vi "数据存储.vi"(10 "字符串":string="E:\\YM\\", 11 "2D data":dbl[][](array[numeric]) caption="二维数据" format="%0.2f") -> ()   [LabVIEW 2013]
uses:
  <vilib>/printing/EasyPrintingControls.llb/report_type.ctl
  <vilib>/printing/EasyPrintingControls.llb/contents.ctl
  <vilib>/Utility/NIReport.llb/NI_report.lvclass
  <vilib>/Utility/file.llb/Write To Spreadsheet File (DBL).vi
  <vilib>/printing/EasyPrinting.llb/Easy Print VI Panel or Documentation (path).vi
  <vilib>/Utility/NIReport.llb/NI_ReportGenerationCore.lvlib
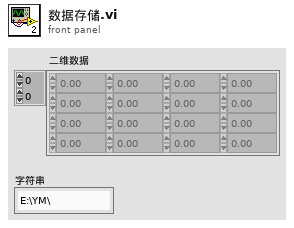
[diagram p1: front panel]
types:
  T1 = typedef "NI_ReportGenerationCore.lvlib/contents.ctl" = u16
  T2 = typedef "NI_ReportGenerationCore.lvlib/report_type.ctl" = u16
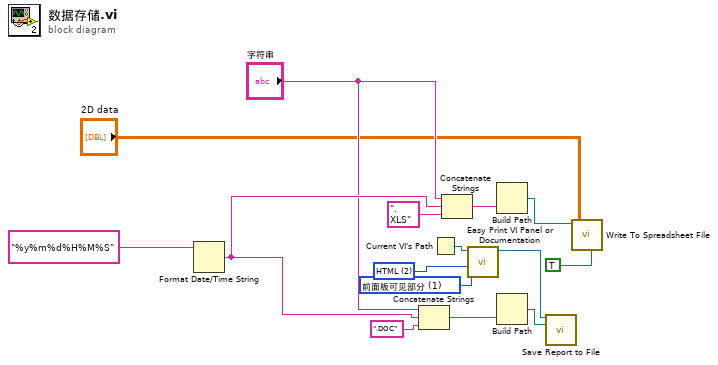
[diagram p0: block diagram]
diagram:
  w3 = T1 1 items=["完整前面板", "前面板可见部分", "图标、说明、前面板和程序框图", "说明信息：使用前面板", "说明信息：作为子VI使用", "说明信息：完整", "说明信息：自定义"] ("contents (complete front panel)")
  w11 = T2 2 items=["快速打印", "标准报表", "HTML", "双字节", "Excel"] ("report type (Quick Print)")
  n1 = Format Date/Time String(time format string (%c)="%y%m%d%H%M%S" ("时间格式字符串(%c)")) -> (date/time string=w6:string)  [unwired: 2 in]
  n2 = Concatenate Strings("字符串", w6, ".DOC" ("产品ID")) -> (w9:string)
  n3 = Current VI's Path() -> (path=w12:path)
  n4 = Concatenate Strings("字符串", w6, ".XLS") -> (w14:string)
  n5 = call-poly <vilib>:"Easy Print VI Panel or Documentation.vi"("report type (Quick Print)"=w11, "contents (complete front panel)"=w3, "VI path"=w12) -> ("report out"=w10:refnum<class "NI_report.lvclass">)  [unwired: 7 in, 1 out]
  n6 = Build Path(name or relative path=w14) -> (appended path=w13:path)  [unwired: 1 in]
  n7 = Build Path(name or relative path=w9) -> (appended path=w1:path)  [unwired: 1 in]
  n8 = call-dynamic "Save Report to File.vi"("report in"=w10, "report file path"=w1) -> ()  [unwired: 12 in, 2 out]
  n9 = call-poly <vilib>:"Write To Spreadsheet File.vi"("transpose? (no:F)"=TRUE, "2D data"="2D data", "file path (dialog if empty)"=w13) -> ()  [unwired: 5 in, 1 out]
